vi "Set Delay.vi"(8 "error in (no error)":errorcluster, 10 "Delay":dbl, 11 "Delay Timer in":refnum<class "Output Timer.lvclass">) -> (0 "error out":errorcluster, 3 "Delay Timer out":refnum<class "Output Timer.lvclass">)   [LabVIEW 2013, in "Output Timer.lvclass"]
uses:
  Output Timer.lvclass
  Output Timer.lvclass/Output Timer.ctl
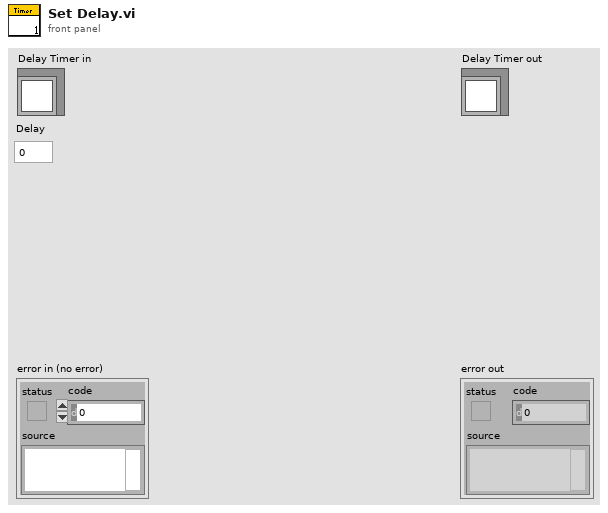
[diagram p1: front panel]
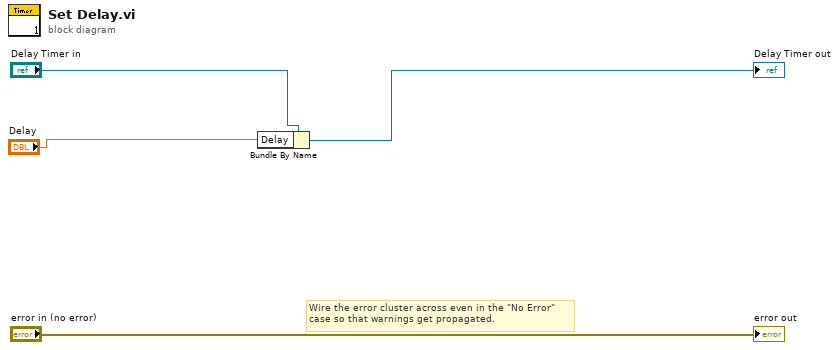
[diagram p0: block diagram]
diagram:
  # "Wire the error cluster across even in the \"No Error\"\ncase so that warnings get propagated."
  n1 = Bundle By Name(cluster="Delay Timer in", "Delay"="Delay") -> (→"Delay Timer out":refnum<class "Output Timer.lvclass">)
  "error out" <- "error in (no error)"
